vi "HEADERS Request.vi"(7 "Header":T1, 8 "error in (no error)":errorcluster, 9 "Single Header Name":string, 10 "Path (after URL)":string, 11 "REST Interface in":refnum<class "REST Interface.lvclass">) -> (0 "error out":errorcluster, 1 "Header Value(s)":string[](array[string]), 2 "Header Name(s)":string[](array[string]), 3 "REST Interface out":refnum<class "REST Interface.lvclass">, 4 "Status Code":u16)   [LabVIEW 2018, in "REST Interface.lvlib" / "REST Interface.lvclass"]
uses:
  REST Interface.lvclass
  Custom Controls/Headers.ctl
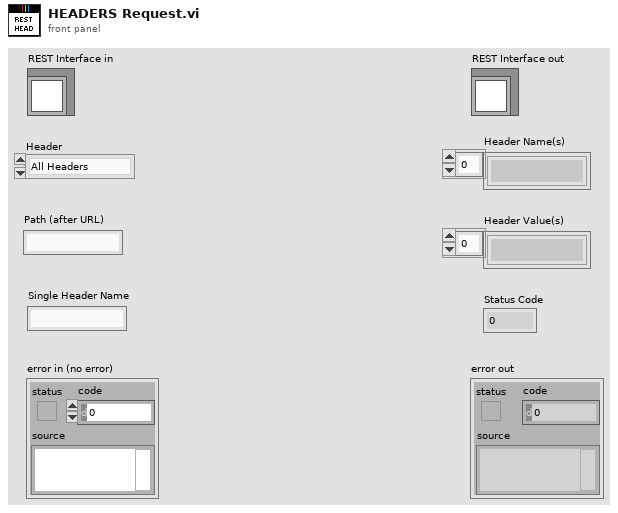
[diagram p1: front panel]
types:
  T1 = typedef "REST Interface.lvlib/REST Interface.lvclass/Headers.ctl" = enum16{"All Headers", "Single Header"}
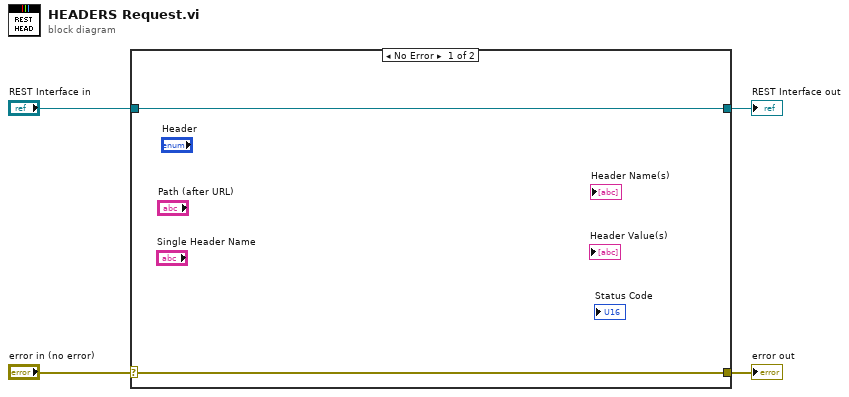
[diagram p0: block diagram]
diagram:
  n1 = case shown="No Error" "error in (no error)" {
    selector: "error in (no error)" -> [w5 w8]
    tunnel: [w5 w8] -> w3
    tunnel: [w6 w7] -> w1
    tunnel: "REST Interface in" -> [w6 w7]
    frame No Error {
    }
    frame Error {
    }
  }
  "error out" <- w3
  "REST Interface out" <- w1
